vi "Digital input.vi"(8 "error in":errorcluster, 11 "DAQmx InPut Setting":T1) -> (0 "error out":errorcluster, 1 "Exit":bool)   [LabVIEW 2015]
uses:
  <vilib>/DAQmx/read.llb/DAQmx Read (Digital 1D Bool 1Chan 1Samp).vi
  <vilib>/DAQmx/create/channels.llb/DAQmx Create Channel (DI-Digital Input).vi
  Galobal variable_TI.vi
  <vilib>/DAQmx/miscellaneous.llb/DAQmx Fill In Error Info.vi
panel:
  in  "Count":i32
  out "Array":bool[](array[boolean])
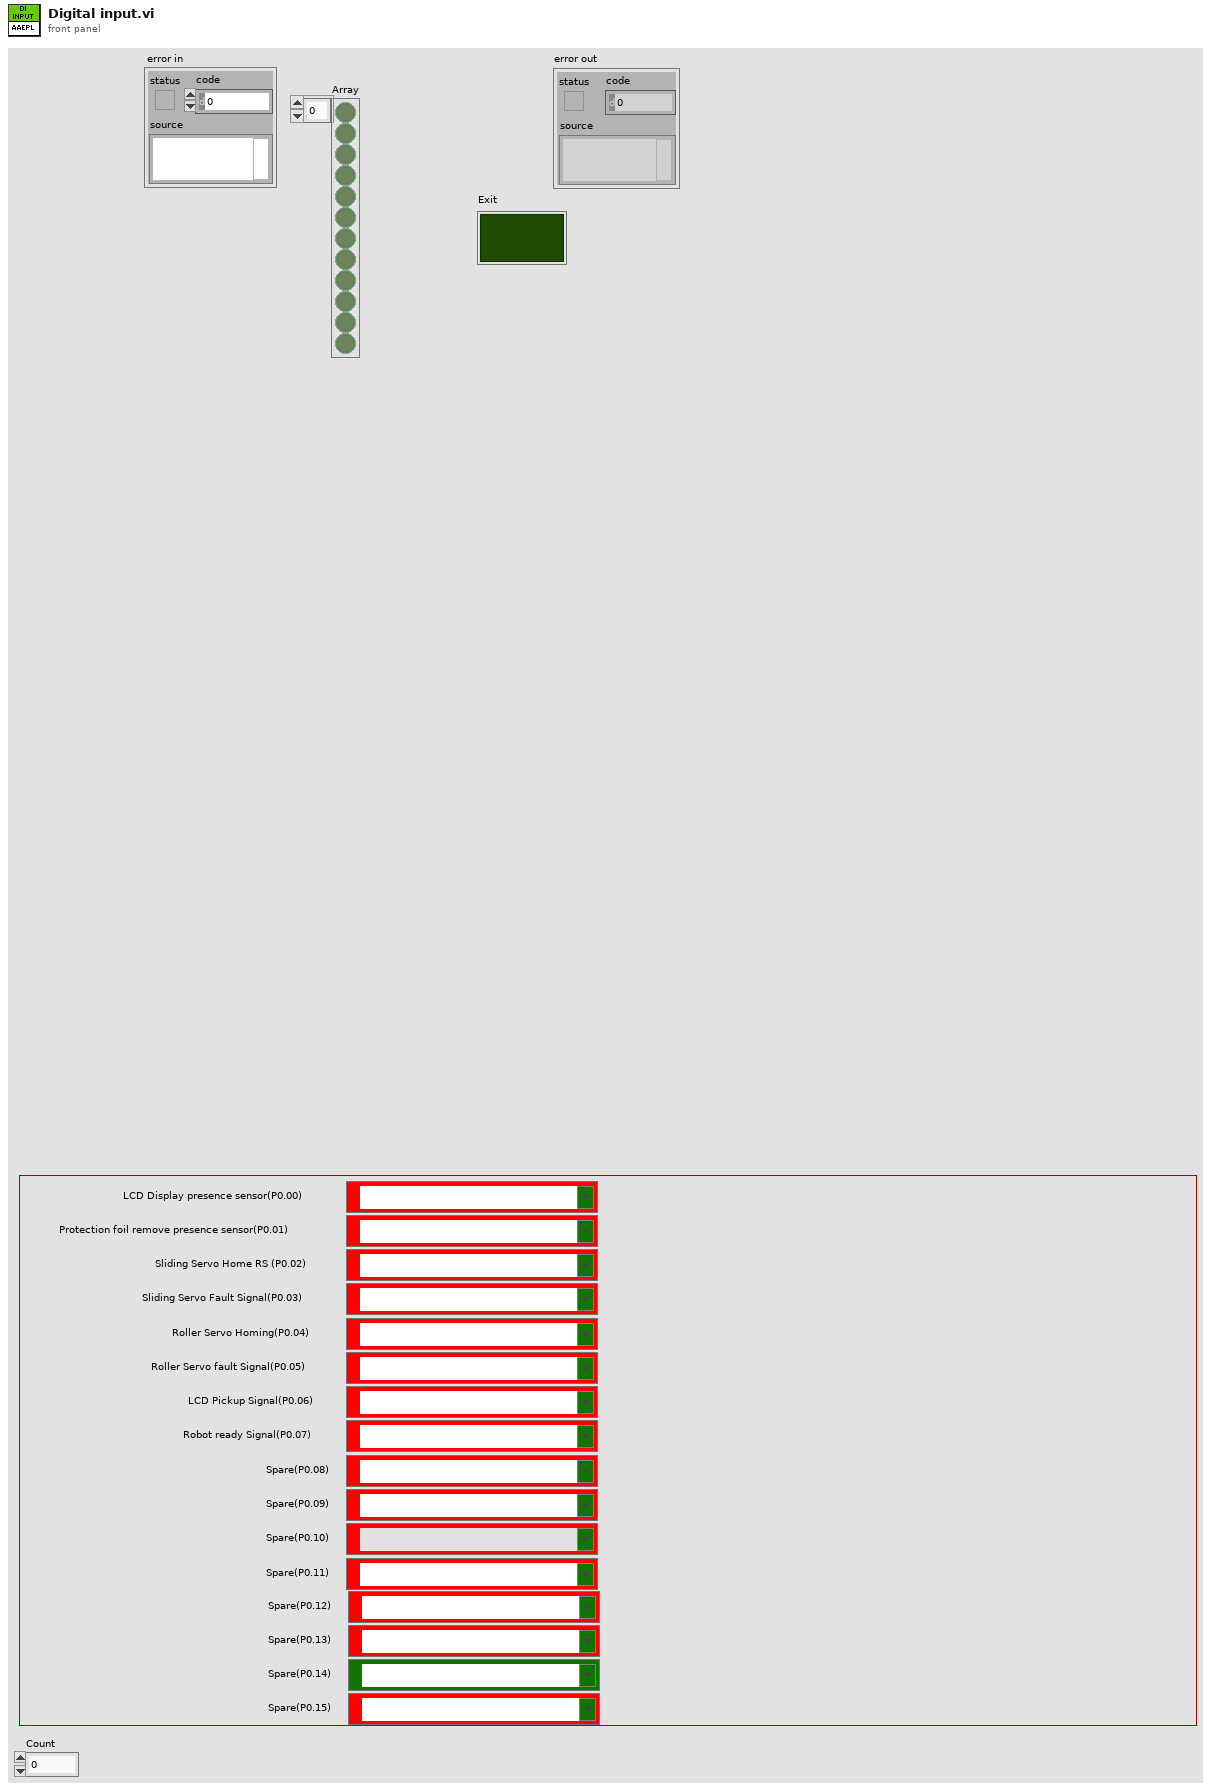
[diagram p1: front panel]
types:
  T1 = cluster{"DAQmx InPut_00":tag, "DAQmx InPut_01":tag, "DAQmx InPut_02":tag, "DAQmx InPut_03":tag, "DAQmx InPut_04":tag, "DAQmx InPut_05":tag, "DAQmx InPut_06":tag, "DAQmx InPut_07":tag, "DAQmx InPut_08":tag, "DAQmx InPut_09":tag, "DAQmx InPut_10":tag, "DAQmx InPut_11":tag, "DAQmx InPut_12":tag, "DAQmx InPut_13":tag, "DAQmx InPut_14":tag, "DAQmx InPut_15":tag}
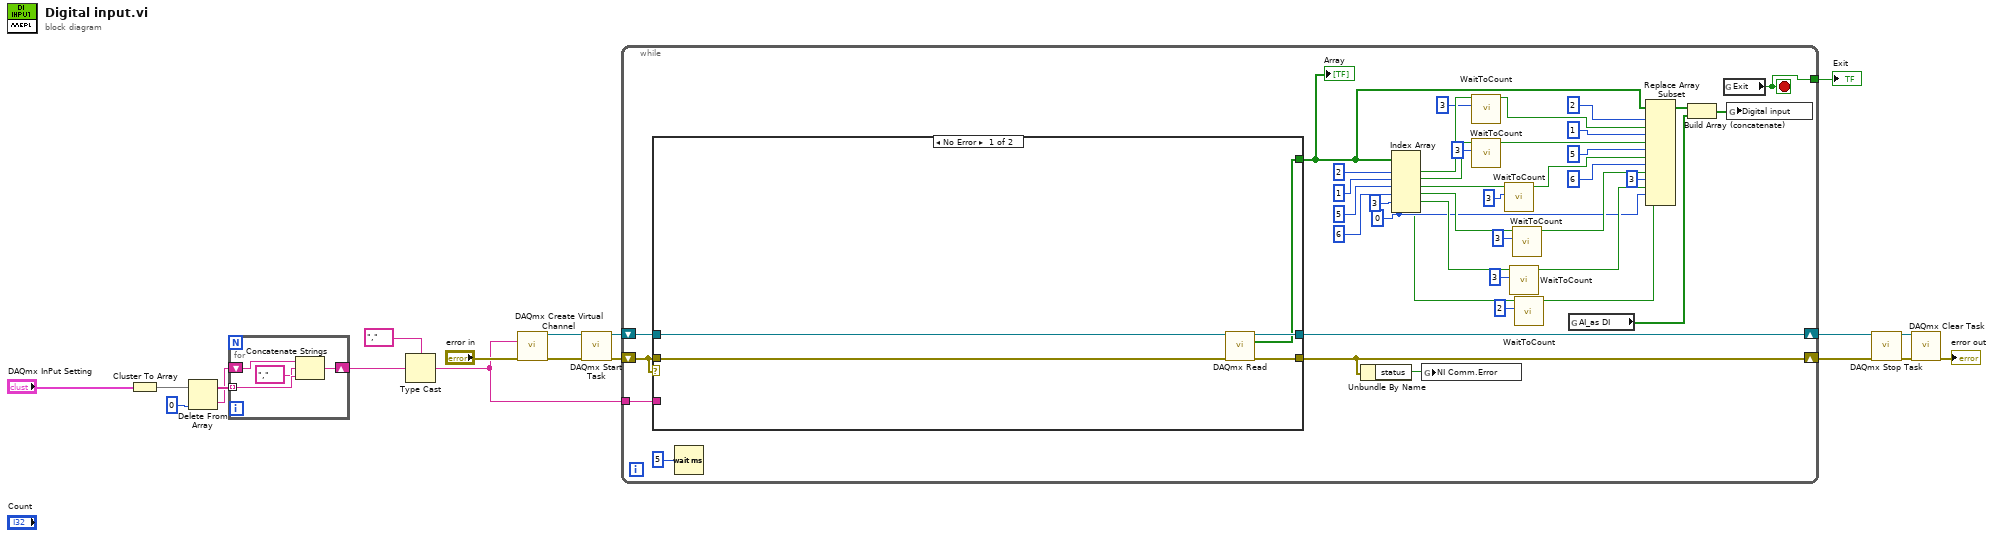
[diagram p0: block diagram]
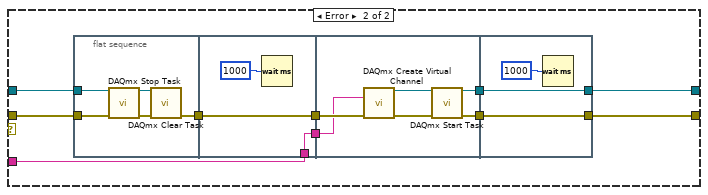
[diagram p2: hidden frame]
diagram:
  n1 = Cluster To Array(cluster="DAQmx InPut Setting") -> (array=w9:tag[])
  n2 = Delete From Array(array=w9, index=0) -> (deleted portion=w6:tag, array with subset deleted=w8:tag[])  [unwired: 1 in]
  n3 = for {
    tunnel: w8 -> [w22] mode=indexing
    shift-right: [w20] -> w4
    shift-left: w6 -> [w23]
    n4 = Concatenate Strings(w23, tag "," ("1."), w22) -> (w20:string)
  }
  n5 = Type Cast(type=tag "," ("1."), x=w4) -> (*(type *) &x=w3:tag)
  n6 = call-poly <vilib>:"DAQmx Create Virtual Channel.vi"("lines"=w3, "error in"="error in") -> ("task out"=w19:refnum<k21>, "error out"=w18:errorcluster)  [unwired: 3 in, 9 out]
  n7 = call <vilib>:"DAQmx Start Task.vi"("task/channels in"=w19, "error in"=w18) -> ("task out"=w16:refnum<k21>, "error out"=w17:errorcluster)  [unwired: 12 out]
  n8 = while {
    shift-right: [w56] -> w13
    shift-left: w17 -> [w64]
    shift-right: [w62] -> w12
    shift-left: w16 -> [w63]
    tunnel: w3 -> [w61]
    tunnel: [w60] -> w10
    stop <- w60 stop-if-true
    w27 = 0 ("index")
    n9 = case shown="No Error" w64 {
      tunnel: w64 -> [w69 w78]
      tunnel: w63 -> [w68 w79]
      tunnel: [w67 w71] -> w56
      tunnel: [w66 w70] -> w62
      tunnel: w61 -> [_ w74]
      tunnel: [w65 _] -> w51
      frame No Error {
        n10 = call-poly <vilib>:"DAQmx Read.vi"("task/channels in"=w68, "error in"=w69) -> ("task out"=w66:refnum<k21>, "data"=w65:bool[], "error out"=w67:errorcluster)  [unwired: 1 in, 10 out]
      }
      frame Error {
        n11 = flat-sequence {
          tunnel: w79 -> [w82]
          tunnel: w78 -> [w81]
          tunnel: [w80] -> w77
          tunnel: w77 -> [w86]
          tunnel: [w86] -> w76
          tunnel: [w85] -> w75
          tunnel: w74 -> [w85]
          tunnel: w76 -> [w91]
          tunnel: w75 -> [w90]
          tunnel: [w89] -> w73
          tunnel: [w88] -> w72
          tunnel: w73 -> [w96]
          tunnel: w72 -> [w95]
          tunnel: [w96] -> w71
          tunnel: [w95] -> w70
          frame #0 {
            n12 = call <vilib>:"DAQmx Stop Task.vi"("task/channels in"=w82, "error in"=w81) -> ("task out"=w83:refnum<k21>, "error out"=w84:errorcluster)  [unwired: 12 in]
            n13 = call <vilib>:"DAQmx Clear Task.vi"("task in"=w83, "error in"=w84) -> ("error out"=w80:errorcluster)  [unwired: 13 in]
          }
          frame #1 {
            n14 = Wait (ms)(milliseconds to wait=u32 1000) -> ()  [unwired: 1 out]
          }
          frame #2 {
            n15 = call-poly <vilib>:"DAQmx Create Virtual Channel.vi"("lines"=w90, "error in"=w91) -> ("task out"=w92:refnum<k21>, "error out"=w93:errorcluster)  [unwired: 3 in, 9 out]
            n16 = call <vilib>:"DAQmx Start Task.vi"("task/channels in"=w92, "error in"=w93) -> ("task out"=w88:refnum<k21>, "error out"=w89:errorcluster)  [unwired: 12 out]
          }
          frame #3 {
            n17 = Wait (ms)(milliseconds to wait=u32 1000) -> ()  [unwired: 1 out]
          }
        }
      }
    }
    "Array" <- w51
    n18 = Wait (ms)(milliseconds to wait=u32 5) -> ()  [unwired: 1 out]
    n19 = Unbundle By Name(w56) -> ("status"=w55:bool)
    n20 = Index Array(array=w51, index #1=2 ("index"), index #2=1 ("index"), index #3=5 ("index"), index #4=6 ("index"), index #5=3 ("index"), index #6=w27) -> (element #1=w54:bool, element #2=w48:bool, element #3=w40:bool, element #4=w39:bool, element #5=w31:bool, element #6=w25:bool)
    n21 = global write "Galobal variable_TI.vi" "NI Comm.Error"(w55) -> ()
    n22 = call "WaitToCount.vi"("Count"=3, "Boolean-01"=w54) -> ("Boolean-01-Indicator"=w52:bool)  [unwired: 8 in, 1 out]
    n23 = call "WaitToCount.vi"("Count"=3, "Boolean-01"=w48) -> ("Boolean-01-Indicator"=w47:bool)  [unwired: 8 in, 1 out]
    n24 = call "WaitToCount.vi"("Count"=3, "Boolean-01"=w40) -> ("Boolean-01-Indicator"=w36:bool)  [unwired: 8 in, 1 out]
    n25 = call "WaitToCount.vi"("Count"=3, "Boolean-01"=w31) -> ("Boolean-01-Indicator"=w29:bool)  [unwired: 8 in, 1 out]
    n26 = call "WaitToCount.vi"("Count"=3, "Boolean-01"=w39) -> ("Boolean-01-Indicator"=w35:bool)  [unwired: 8 in, 1 out]
    n27 = call "WaitToCount.vi"("Count"=2, "Boolean-01"=w25) -> ("Boolean-01-Indicator"=w24:bool)  [unwired: 8 in, 1 out]
    n28 = global read "Galobal variable_TI.vi" "AI_as DI"() -> (w58:bool[])
    n29 = Replace Array Subset(array=w51, new element #1=w52, index #1=2 ("index"), new element #2=w47, index #2=1 ("index"), new element #3=w36, index #3=5 ("index"), new element #4=w35, index #4=6 ("index"), new element #5=w29, index #5=3 ("index"), new element #6=w24, index #6=w27) -> (w50:bool[])
    n30 = Build Array (concatenate)(w50, w58) -> (w59:bool[])
    n31 = global read "Galobal variable_TI.vi" "Exit"() -> (w60:bool)
    n32 = global write "Galobal variable_TI.vi" "Digital input"(w59) -> ()
  }
  "Exit" <- w10
  n33 = call <vilib>:"DAQmx Stop Task.vi"("task/channels in"=w12, "error in"=w13) -> ("task out"=w14:refnum<k21>, "error out"=w15:errorcluster)  [unwired: 12 in]
  n34 = call <vilib>:"DAQmx Clear Task.vi"("task in"=w14, "error in"=w15) -> ("error out"=→"error out":errorcluster)  [unwired: 13 in]
